vi "Instrument_IP_Address2.vi"(11 "Instrument":T1(ring)=enum."spoldrx") -> (2 "Port":u16, 3 "IP Address":string="0.0.0.0")   [LabVIEW 2012]
doc: "Returns the IP address and port of ATE instruments"
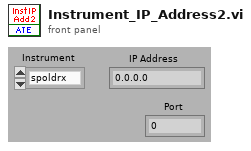
[diagram p1: front panel]
types:
  T1 = enum16{"N1911A", "Siggen", "34980a", "E4418B", "Rvp8", "spoldrx"}
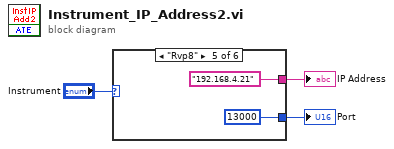
[diagram p0: block diagram]
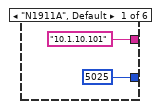
[diagram p2: hidden frame]
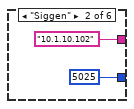
[diagram p3: hidden frame]
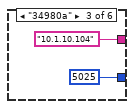
[diagram p4: hidden frame]
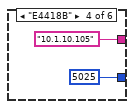
[diagram p5: hidden frame]
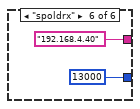
[diagram p6: hidden frame]
diagram:
  n1 = case shown="\"Rvp8\"" "Instrument" {
    tunnel: ["10.1.10.101" "10.1.10.102" "10.1.10.104" "10.1.10.105" "192.168.4.21" "192.168.4.40"] -> w2
    tunnel: [5025 5025 5025 5025 13000 13000] -> w1
    frame "N1911A", Default {
    }
    frame "Siggen" {
    }
    frame "34980a" {
    }
    frame "E4418B" {
    }
    frame "Rvp8" {
    }
    frame "spoldrx" {
    }
  }
  "IP Address" <- w2
  "Port" <- w1
